vi "tcs shm put Sample Timestamp LV.vi"(8 "error in (no error)":errorcluster, 11 "Timestamp_Ctl":cluster{"size":i32, "data":string}) -> (0 "error out":errorcluster, 2 "function return":i32, 3 "Timestamp_Ctl out":cluster{"size":i32, "data":string})   [LabVIEW 2016, in "SALLV_tcs.lvlib"]
doc: "int tcs_shm_putSample_TimestampLV(tcs_TimestampLV *Timestamp_Ctl );"
uses:
  SALLV_tcs.lvlib
  SALLV_tcs.so
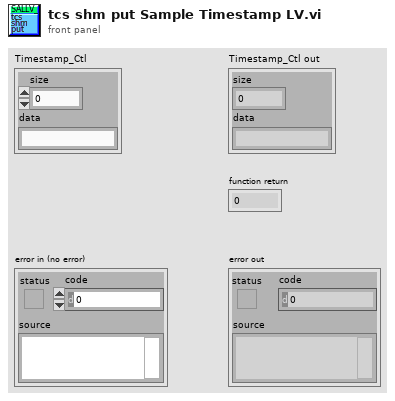
[diagram p1: front panel]
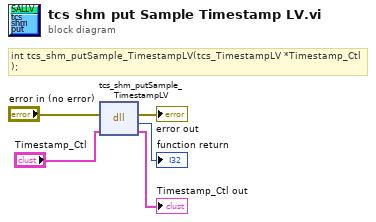
[diagram p0: block diagram]
diagram:
  # "int tcs_shm_putSample_TimestampLV(tcs_TimestampLV *Timestamp_Ctl );"
  n1 = dll-call lib="home/plotz/SALLV_tcs/SALLV_tcs.*" fn="tcs_shm_putSample_TimestampLV"(error in="error in (no error)", "Timestamp_Ctl"="Timestamp_Ctl") -> (error out=→"error out":errorcluster, →"function return":i32, "Timestamp_Ctl"=→"Timestamp_Ctl out":cluster{"size":i32, "data":string})  [unwired: 2 in, 1 out]
